vi "Texte in VIs uebersetzen.vi"(0 "Sprachliste":string[][](array[string]), 5 "String-Array zum Übersetzen":string[](array[string]), 7 "2D String-Array zum Übersetzen":string[][](array[string]), 9 "String zum Übersetzen":string, 11 "error in (no error)":errorcluster caption="Fehler (Eingang, kein Fehler)") -> (4 "Sprachliste out":string[][](array[string]), 6 "String-Array zum Übersetzen":string[](array[string]), 8 "2D String-Array zum Übersetzen":string[][](array[string]), 10 "String zum Übersetzen":string, 15 "error out":errorcluster caption="Fehler (Ausgang)")   [LabVIEW 2020, in "Sprachverwaltung.lvlib"]
uses:
  Sprachverwaltung.lvlib
  Seiten/System Einstellungen V2/System Einstellungen V2.lvlib
  Seiten/System Einstellungen V2/Aktioen FGV System Konstanten.ctl
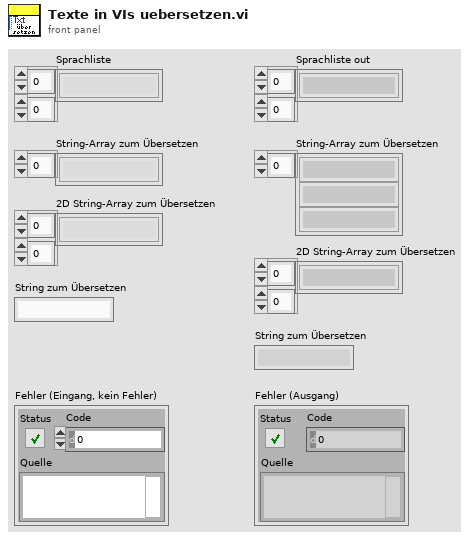
[diagram p1: front panel]
types:
  T1 = typedef "System Einstellungen V2.lvlib/Aktioen FGV System Konstanten.ctl" = enum16{"lesen", "laden", "speichern", "Sprache"}
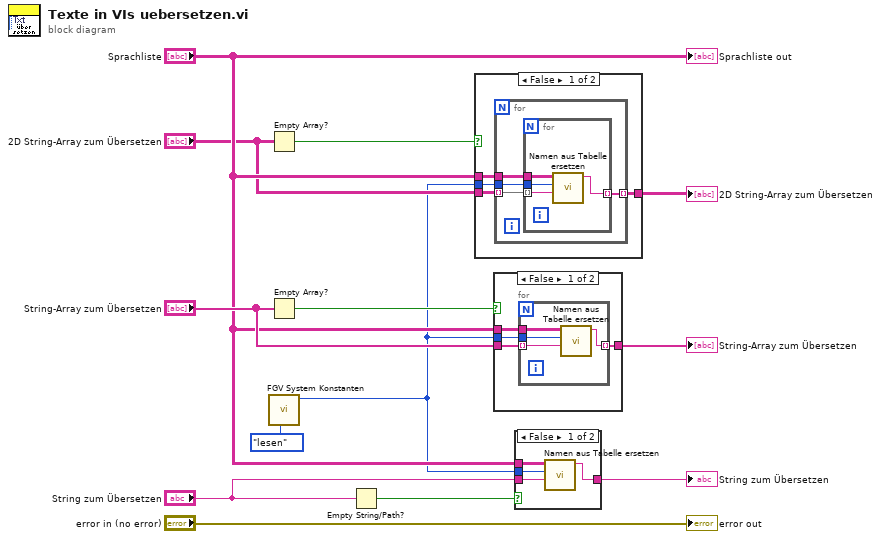
[diagram p0: block diagram]
diagram:
  n1 = Empty Array?(array="2D String-Array zum Übersetzen") -> (empty?=w5:bool)
  n2 = Empty Array?(array="String-Array zum Übersetzen") -> (empty?=w7:bool)
  n3 = call "FGV System Konstanten.vi"("Aktionen"=Aktioen_FGV_System_Konstanten."lesen") -> ("Sprachindex"=w1:u16)  [unwired: 6 in, 4 out]
  n4 = Empty String/Path?(string/path="String zum Übersetzen") -> (empty?=w12:bool)
  n5 = case shown="False" w5 {
    tunnel: "Sprachliste" -> [w17 _]
    tunnel: w1 -> [w16 _]
    tunnel: [w15 w26] -> w2
    tunnel: "2D String-Array zum Übersetzen" -> [w14 w26]
    frame False {
      n6 = for {
        tunnel: w17 -> [w21]
        tunnel: w16 -> [w20]
        tunnel: [w19] -> w15 mode=indexing
        tunnel: w14 -> [w18] mode=indexing
        n7 = for {
          tunnel: w21 -> [w25]
          tunnel: w20 -> [w24]
          tunnel: [w22] -> w19 mode=indexing
          tunnel: w18 -> [w23] mode=indexing
          n8 = call "Namen aus Tabelle ersetzen.vi"("Regulärer Ausdruck"=w23, "Sprachauswahl"=w24, "Tabelle"=w25) -> ("Übersetzung"=w22:string)  [unwired: 7 in, 1 out]
        }
      }
    }
    frame True {
    }
  }
  "2D String-Array zum Übersetzen" <- w2
  n9 = case shown="False" w7 {
    tunnel: "Sprachliste" -> [w30 _]
    tunnel: w1 -> [w29 _]
    tunnel: [w28 w35] -> w10
    tunnel: "String-Array zum Übersetzen" -> [w27 w35]
    frame False {
      n10 = for {
        tunnel: w30 -> [w34]
        tunnel: w29 -> [w33]
        tunnel: [w31] -> w28 mode=indexing
        tunnel: w27 -> [w32] mode=indexing
        n11 = call "Namen aus Tabelle ersetzen.vi"("Regulärer Ausdruck"=w32, "Sprachauswahl"=w33, "Tabelle"=w34) -> ("Übersetzung"=w31:string)  [unwired: 7 in, 1 out]
      }
    }
    frame True {
    }
  }
  "String-Array zum Übersetzen" <- w10
  n12 = case shown="False" w12 {
    tunnel: "Sprachliste" -> [w39 _]
    tunnel: w1 -> [w38 _]
    tunnel: "String zum Übersetzen" -> [w37 w40]
    tunnel: [w36 w40] -> w9
    frame False {
      n13 = call "Namen aus Tabelle ersetzen.vi"("Regulärer Ausdruck"=w37, "Sprachauswahl"=w38, "Tabelle"=w39) -> ("Übersetzung"=w36:string)  [unwired: 7 in, 1 out]
    }
    frame True {
    }
  }
  "String zum Übersetzen" <- w9
  "error out" <- "error in (no error)"
  "Sprachliste out" <- "Sprachliste"
